vi "coordinates for simulation.vi"(0 "phi1":dbl, 5 "k1":dbl, 9 "phi2":dbl, 11 "k2":dbl, 12 "s1":dbl, 14 "s2":dbl) -> (4 "X":dbl[](array[numeric]), 8 "Y":dbl[](array[numeric]), 15 "Z":dbl[](array[numeric]))   [LabVIEW 2017]
uses:
  <vilib>/imath/engines/lvmath2/RunTimeEngine/Managers/WorkSpace/UID Generator.vi
  <vilib>/imath/engines/lvmath2/RunTimeEngine/RunTimeType/NIMS_RunTimeType_From StrictType (excl LVString).vi
  <instcachedir>/0/NIMS_RunTimeType_From StrictType (excl LVString)_1019F277F0A747EDBCA0F6C52CA54500.lvgen/NIMS_RunTimeType_From StrictType (excl LVString)_1019F277F0A747EDBCA0F6C52CA54500_000.vi
  <vilib>/imath/engines/lvmath2/RunTimeEngine/LocalVariableDefStatement/MC_LocalVariableDefStatement_Display.vi
  <vilib>/imath/engines/lvmath2/RunTimeEngine/Managers/SymbolTable/Clear UID.vi
  <vilib>/imath/engines/lvmath2/RunTimeEngine/NodeEndStatement/NIMS_NodeEndStatement_Output.vi
  <instcachedir>/0/NIMS_NodeEndStatement_Output_53EC0D466D134D7ABD903AC30B43404B.lvgen/NIMS_NodeEndStatement_Output_53EC0D466D134D7ABD903AC30B43404B_001.vi
  <vilib>/imath/engines/lvmath2/RunTimeEngine/ErrorHandling/NIMS_Finalize Error.vi
  <vilib>/imath/engines/lvmath2/RunTimeEngine/Managers/SymbolTable/NIMS_WorkSpace.lvlib
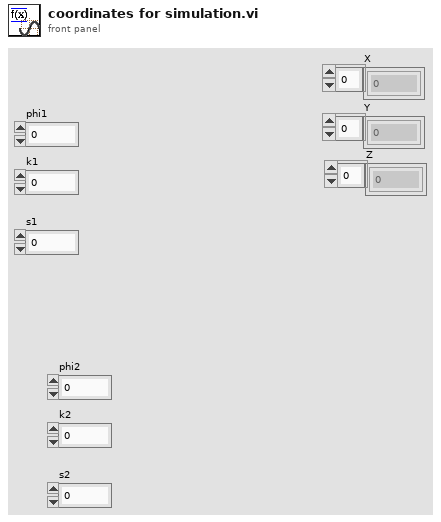
[diagram p1: front panel]
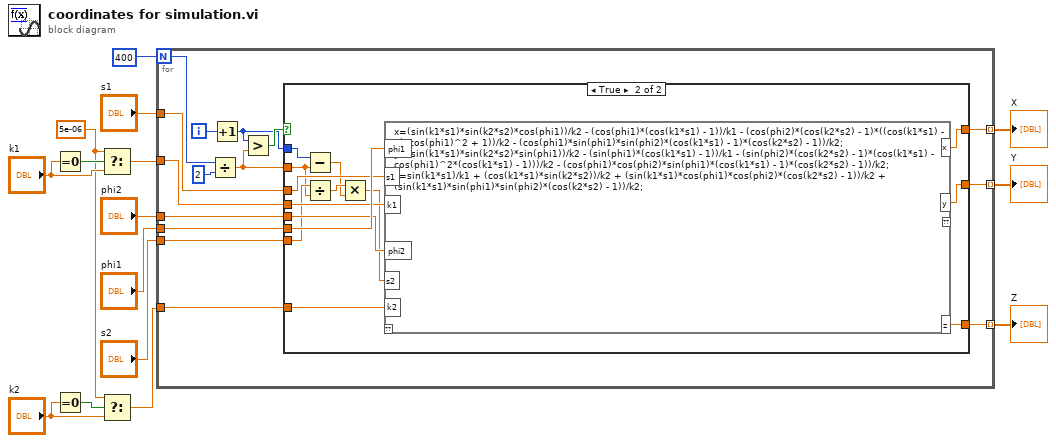
[diagram p0: block diagram]
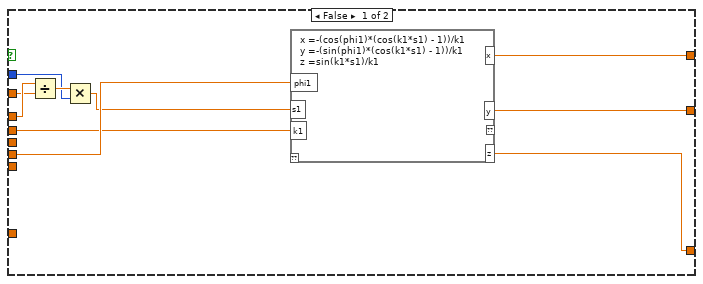
[diagram p2: hidden frame]
diagram:
  w3 = 5e-06
  n1 = Equal To 0?(x="k1") -> (x = 0?=w5:bool)
  n2 = Equal To 0?(x="k2") -> (x = 0?=w7:bool)
  n3 = Select(t=w3, s=w5, f="k1") -> (s? t:f=w1:dbl)
  n4 = Select(t=w3, s=w7, f="k2") -> (s? t:f=w2:dbl)
  n5 = for {
    N: 400 -> [w21]
    tunnel: [w30] -> w14 mode=indexing
    tunnel: [w29] -> w13 mode=indexing
    tunnel: [w28] -> w12 mode=indexing
    tunnel: "phi1" -> [w27]
    tunnel: "s1" -> [w22]
    tunnel: w1 -> [w26]
    tunnel: "phi2" -> [w18]
    tunnel: w2 -> [w17]
    tunnel: "s2" -> [w16]
    i -> [w24]
    n6 = Divide(x=w21, y=2) -> (x/y=w19:dbl)
    n7 = Increment(x=w24) -> (x+1=w20:i32)
    n8 = Greater?(x=w20, y=w19) -> (0:w23:bool)
    n9 = case shown="True" w23 {
      tunnel: [w38 w148] -> w30
      tunnel: [w37 w147] -> w29
      tunnel: [w36 w146] -> w28
      tunnel: w27 -> [w40 w145]
      tunnel: w26 -> [w39 w143]
      tunnel: w22 -> [w35 w144]
      tunnel: w20 -> [w33 w137]
      tunnel: w19 -> [w31 w135]
      tunnel: w18 -> [_ w142]
      tunnel: w17 -> [_ w141]
      tunnel: w16 -> [_ w140]
      frame False {
        n10 = Divide(x=w35, y=w31) -> (x/y=w34:dbl)
        n11 = Multiply(x=w34, y=w33) -> (x*y=w32:dbl)
        n12 = mathscript code="x =-(cos(phi1)*(cos(k1*s1) - 1))/k1\ny =-(sin(phi1)*(cos(k1*s1) - 1))/k1\nz =sin(k1*s1)/k1"("phi1"=w40, "s1"=w32, "k1"=w39) -> ("x"=w38:dbl, "y"=w37:dbl, "z"=w36:dbl)  [unwired: 1 in, 1 out]
      }
      frame True {
        n13 = Subtract(x=w137, y=w135) -> (x-y=w136:dbl)
        n14 = Divide(x=w140, y=w135) -> (x/y=w139:dbl)
        n15 = Multiply(x=w139, y=w136) -> (x*y=w138:dbl)
        n16 = mathscript code="x=(sin(k1*s1)*sin(k2*s2)*cos(phi1))/k2 - (cos(phi1)*(cos(k1*s1) - 1))/k1 - (cos(phi2)*(cos(k2*s2) - 1)*((cos(k1*s1) - 1)*cos(phi1)^2 + 1))/k2 - (cos(phi1)*sin(phi1)*sin(phi2)*(cos(k1*s1) - 1)*(cos(k2*s2) - 1))/k2;\ny=(sin(k1*s1)*sin(k2*s2)*sin(phi1))/k2 - (sin(phi1)*(cos(k1*s1) - 1))/k1 - (sin(phi2)*(cos(k2*s2) - 1)*(cos(k1*s1) - cos(phi1)^2*(cos(k1*s1) - 1)))/k2 - (cos(phi1)*cos(phi2)*sin(phi1)*(cos(k1*s1) - 1)*(cos(k2*s2) - 1))/k2;\nz=sin(k1*s1)/k1 + (cos(k1*s1)*sin(k2*s2))/k2 + (sin(k1*s1)*cos(phi1)*cos(phi2)*(cos(k2*s2) - 1))/k2 + (sin(k1*s1)*sin(phi1)*sin(phi2)*(cos(k2*s2) - 1))/k2;"("phi1"=w145, "s1"=w144, "k1"=w143, "phi2"=w142, "s2"=w138, "k2"=w141) -> ("x"=w148:dbl, "y"=w147:dbl, "z"=w146:dbl)  [unwired: 1 in, 1 out]
      }
    }
  }
  "X" <- w14
  "Y" <- w13
  "Z" <- w12
